vi "EndTestSuite.vi"(8 "error in (no error)":errorcluster, 10 "TestSuite":refnum<class "TestSuite.lvclass">, 11 "TestResult in":refnum<class "TestResult.lvclass">) -> (0 "error out":errorcluster, 3 "TestResult out":refnum<class "TestResult.lvclass">)   [LabVIEW 2019, in "TestResult.lvclass"]
uses:
  TestResult.lvclass
  TestSuite/TestSuite.lvclass
  TestResult.lvclass/TestResult.ctl
  TestListener/TestListener.lvclass
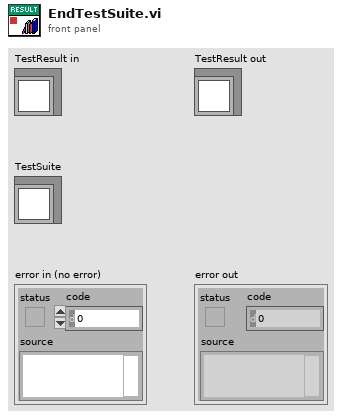
[diagram p1: front panel]
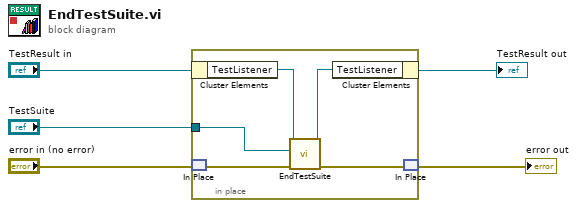
[diagram p0: block diagram]
diagram:
  n1 = in-place {
    in-place-border: "TestSuite" -> [w10]
    n2 = in-place-cluster #1("TestResult in") -> ("TestListener"=w7:refnum<class "TestListener.lvclass">)
    n3 = in-place-match #2("error in (no error)") -> (w9:errorcluster)
    n4 = call-dynamic "EndTestSuite.vi"("error in (no error)"=w9, "TestSuite"=w10, "TestListener in"=w7) -> ("error out"=w8:errorcluster, "TestListener out"=w6:refnum<class "TestListener.lvclass">)  [unwired: 7 in]
    n5 = in-place-cluster #1("TestListener"=w6) -> (→"TestResult out":refnum<class "TestResult.lvclass">)
    n6 = in-place-match #2(w8) -> (→"error out":errorcluster)
  }
